vi "NI_event_scope.vi"() -> ()   [LabVIEW 2024]
uses:
  D:/git/Sourcegrid-LabVIEW/dll/SourceGrid.dll
  dll/SourceGrid.dll
  MyEventGrid/MyEventGrid.lvclass
  D:/git/Sourcegrid-LabVIEW/source/Grid/SourceGrid.lvclass
  MyEventGrid/MyEventGrid.lvclass/MyEventGrid.ctl
  source/Grid/SourceGrid.lvclass
  source/Cells/Cell Context/Cell Context.lvclass
  <vilib>/Utility/Data Type/NI_Data Type.lvlib
  <vilib>/Utility/Data Type/Type Definitions/Data Type.ctl
panel:
  in  "stop":bool
  out "onValueChanged Value":variant
  out "onValueChanged Value type":T1
  out "onClick Position":string
  out "onClick Value":variant
  in  "Grid Container":refnum<k24>(container)
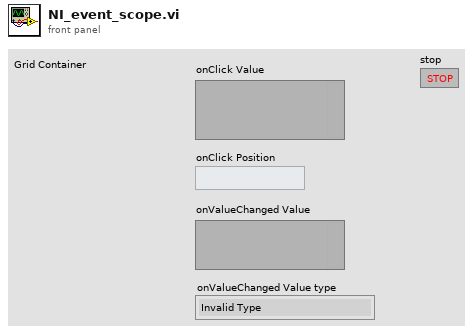
[diagram p1: front panel]
types:
  T1 = typedef "NI_Data Type.lvlib/Data Type.ctl" = enum8{"Invalid Type", "Void", "I8", "I16", "I32", "I64", "U8", "U16", "U32", "U64", "Single Float", "Double Float", "Extended Float", "Single Complex", "Double Complex", "Extended Complex", "Enum U8", "Enum U16", "Enum U32", "Enum U64", "Single Float With Unit", "Double Float With Unit", "Extended Float With Unit", "Single Complex with Unit", "Double Complex with Unit", "Extended Complex with Unit", "Boolean", "String", "Path", "Picture", "Tag", "Array", "Cluster", "Variant", "LV Variant", "Waveform", "Timestamp", "Digital Waveform", "Digital Data", "ExpressData", "Refnum", "External Data", "VI", "Poly VI", "LabVIEW Class Instance", "Fixed Point", "Set Collection", "Map Collection"}
  T2 = cluster{"onClick":refnum<user-event>, "onDoubleClick":refnum<user-event>, "onValueChanged":refnum<user-event>}
  T3 = typedef "Rendezvous RefNum" = refnum<k1>
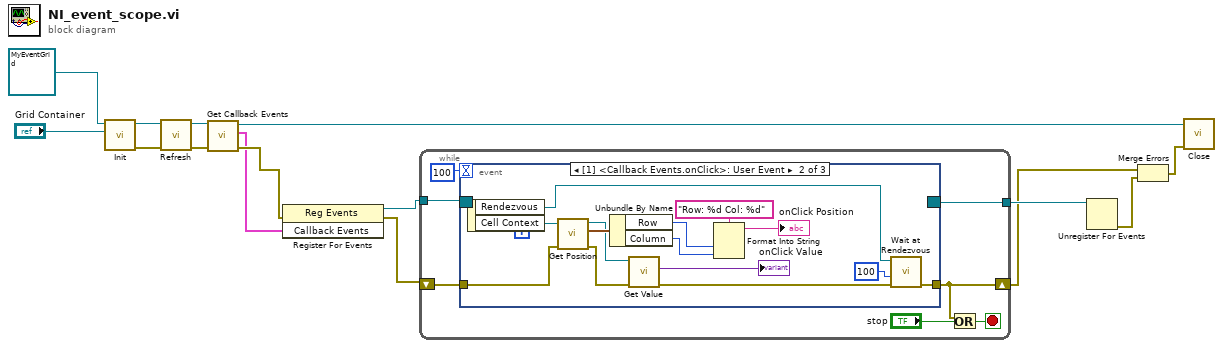
[diagram p0: block diagram]
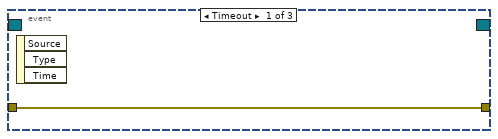
[diagram p2: hidden frame]
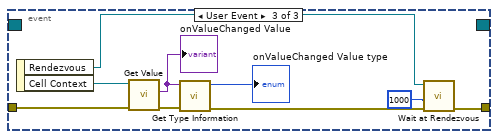
[diagram p3: hidden frame]
diagram:
  n1 = call-dynamic "Init.vi"("Sourcegrid Container"="Grid Container", "MyEventGrid in"=refnum<class "MyEventGrid.lvclass"> refnum ("Grid in")) -> ("error out"=w11:errorcluster, "MyEventGrid out"=w10:refnum<class "MyEventGrid.lvclass">)  [unwired: 8 in]
  n2 = call "Refresh.vi"("error in"=w11, "SourceGrid in"=w10) -> ("error out"=w12:errorcluster, "SourceGrid out"=w9:refnum<class "MyEventGrid.lvclass">)  [unwired: 8 in]
  n3 = call "Get Callback Events.vi"("MyEventGrid in"=w9) -> ("Callback Events"=w7:T2, "MyEventGrid out"=w8:refnum<class "MyEventGrid.lvclass">)  [unwired: 9 in]
  n4 = register-events(error in=w12, w7) -> (reference out=w5:refnum<event-registration>, error out=w4:errorcluster)  [unwired: 1 in]
  n5 = while {
    tunnel: w5 -> [w20]
    tunnel: [w19] -> w6
    shift-right: [w16] -> w1
    shift-left: w4 -> [w15]
    stop <- w17 stop-if-true
    n6 = event shown="[1] <Callback Events.onClick>: User Event" {
      selector: w20 -> [_ _ _]
      dyn-events: [_ _ _] -> w19
      timeout: 100 -> [_ _ _]
      tunnel: [w22 w26 w37] -> w16
      tunnel: w15 -> [w22 w29 w44]
      event Timeout {
        n7 = event-data() -> ()  [unwired: 1 in, 3 out]
      }
      event User Event {
        n8 = event-data() -> ("Rendezvous"=w25:T3, "Cell Context"=w36:refnum<class "Cell Context.lvclass">)  [unwired: 1 in]
        n9 = call "Get Position.vi"("error in"=w29, "Cell Context in"=w36) -> ("error out"=w30:errorcluster, "Position"=w35:cluster{"Row":i32, "Column":i32}, "Cell Context out"=w28:refnum<class "Cell Context.lvclass">)  [unwired: 7 in]
        n10 = Unbundle By Name(w35) -> ("Row"=w32:i32, "Column"=w31:i32)
        n11 = call "Get Value.vi"("error in (no error)"=w30, "Cell Context in"=w28) -> ("error out"=w24:errorcluster, "Value"=→"onClick Value":variant)  [unwired: 7 in, 1 out]
        n12 = Format Into String(format string="Row: %d Col: %d", w32, w31) -> (resulting string=→"onClick Position":string)  [unwired: 2 in, 1 out]
        n13 = call <vilib>:"Wait at Rendezvous.vi"("error in (no error)"=w24, "ms timeout (-1)"=100, "rendezvous"=w25) -> ("error out"=w26:errorcluster)  [unwired: 2 in, 2 out]
      }
      event User Event {
        n14 = event-data() -> ("Rendezvous"=w40:T3, "Cell Context"=w45:refnum<class "Cell Context.lvclass">)  [unwired: 1 in]
        n15 = call "Get Value.vi"("error in (no error)"=w44, "Cell Context in"=w45) -> ("error out"=w42:errorcluster, "Value"=w43:variant)  [unwired: 7 in, 1 out]
        "onValueChanged Value" <- w43
        n16 = call <vilib>:"Get Type Information.vi"("error in (no error)"=w42, "variant"=w43) -> ("error out"=w39:errorcluster, "type"=→"onValueChanged Value type":T1)  [unwired: 5 in, 3 out]
        n17 = call <vilib>:"Wait at Rendezvous.vi"("error in (no error)"=w39, "ms timeout (-1)"=1000, "rendezvous"=w40) -> ("error out"=w37:errorcluster)  [unwired: 2 in, 2 out]
      }
    }
    n18 = Or(x=w16, y="stop") -> (x .or. y?=w17:bool)
  }
  n19 = Unregister For Events(event registration refnum=w6) -> (error out=w2:errorcluster)  [unwired: 1 in]
  n20 = Merge Errors(w1, w2) -> (w3:errorcluster)
  n21 = call-dynamic "Close.vi"("error in"=w3, "MyEventGrid in"=w8) -> ()  [unwired: 8 in, 2 out]
